vi "Stabilization status update.vi"(11 "Color Parameters":T1 {"Color Values"."v'" format="%#_5g"; "Color Values"."Duv" format="%#_5g"; "Color Values"."u'" format="%#_5g"; "Color Values"."CRI" format="%#_5g"; "Color Values"."CCT" format="%#_5g"; "Color Values"."luminousFlux" format="%#_5g"; "R values" format="%#_4g"; "Tristimulus \nValues"."Z" format="%#_5g"; "Tristimulus \nValues"."Y" format="%#_5g"; "Tristimulus \nValues"."X" format="%#_5g"; "Chromaticity \nCoordinates"."v" format="%#_5g"; "Chromaticity \nCoordinates"."u" format="%#_5g"; "Chromaticity \nCoordinates"."z" format="%#_5g"; "Chromaticity \nCoordinates"."y" format="%#_5g"; "Chromaticity \nCoordinates"."x" format="%#_5g"}) -> (2 "luminousFlux":dbl, 3 "Status String":string)   [LabVIEW 2014, in "Timing and Stabilization.lvlib"]
uses:
  avantesSpectrometer/Acquisition/AvaSpec Color Parameters.ctl
  avantesSpectrometer/Acquisition/Sphere Indicator.ctl
  Timing and Stabilization.lvlib
  avantesSpectrometer/AvaSpec.lvlib
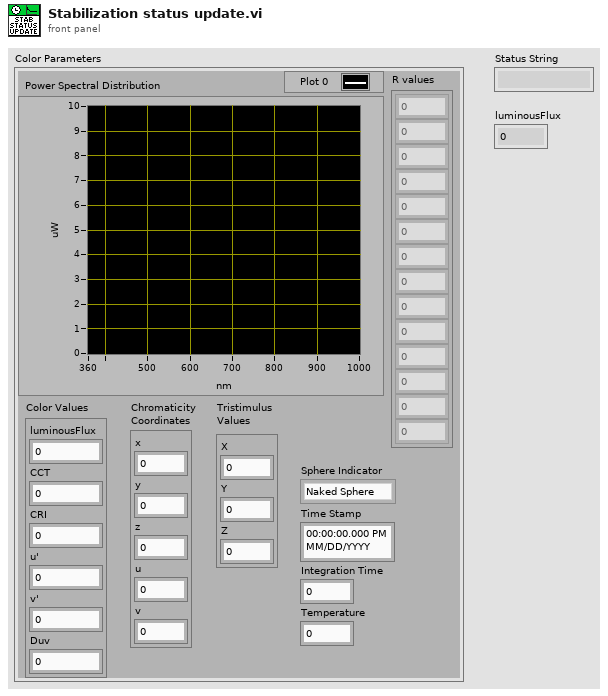
[diagram p1: front panel]
types:
  T1 = typedef "AvaSpec.lvlib/AvaSpec Color Parameters.ctl" = cluster{"Power Spectral Distribution":cluster{"X":dbl, "Y":dbl}[], "Color Values":cluster{"luminousFlux":dbl, "CCT":dbl, "CRI":dbl, "u'":dbl, "v'":dbl, "Duv":dbl}, "R values":dbl[], "Chromaticity \nCoordinates":cluster{"x":dbl, "y":dbl, "z":dbl, "u":dbl, "v":dbl}, "Tristimulus \nValues":cluster{"X":dbl, "Y":dbl, "Z":dbl}, "Time Stamp":timestamp, "Temperature":dbl, "Integration Time":dbl, "Sphere Indicator":T2}
  T2 = typedef "AvaSpec.lvlib/Sphere Indicator.ctl" = enum16{"Naked Sphere", "Insulated Sphere"}
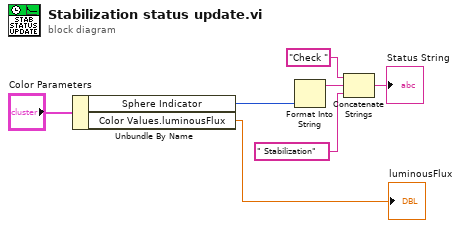
[diagram p0: block diagram]
diagram:
  n1 = Unbundle By Name("Color Parameters") -> ("Sphere Indicator"=w2:T2, "Color Values.luminousFlux"=→"luminousFlux":dbl)
  n2 = Format Into String(w2) -> (resulting string=w3:string)  [unwired: 3 in, 1 out]
  n3 = Concatenate Strings("Check " ("Message"), w3, " Stabilization" ("Message")) -> (→"Status String":string)
